vi "Write Device.vi"(8 "error in":errorcluster, 10 "Device":string, 11 "Config in":refnum<class "Config.lvclass">) -> (0 "error out":errorcluster, 3 "Config out":refnum<class "Config.lvclass">)   [LabVIEW 2023, in "Config.lvlib" / "Config.lvclass"]
doc: "Select device from list of devices and read all key labels and values for the device"
uses:
  Config.lvclass
  Config.lvclass/Config.ctl
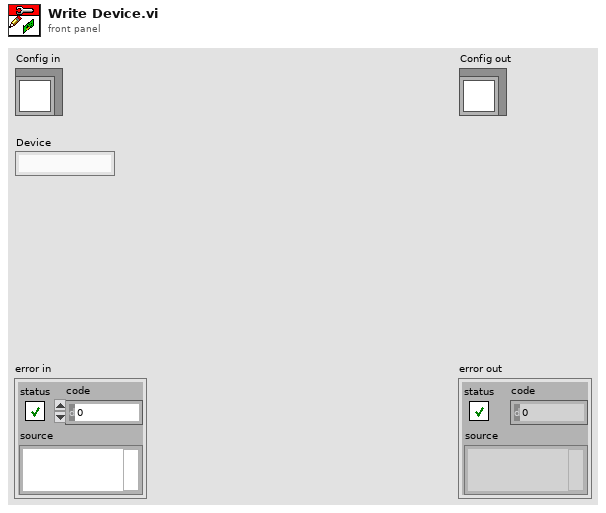
[diagram p1: front panel]
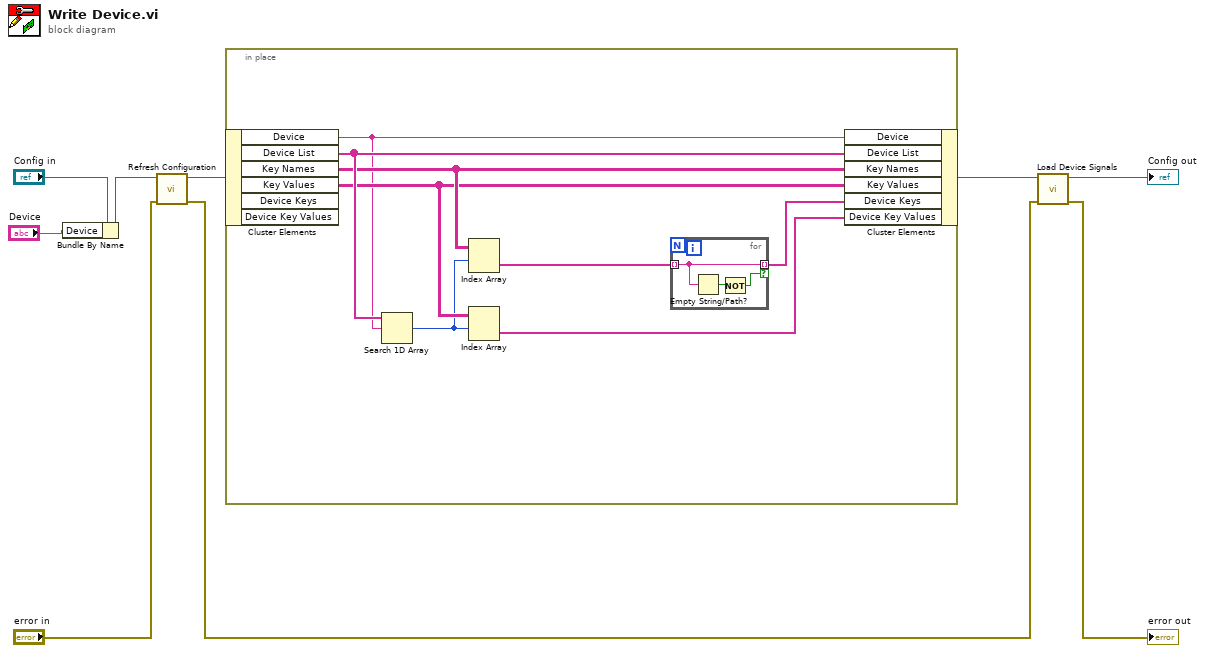
[diagram p0: block diagram]
diagram:
  n1 = Bundle By Name(cluster="Config in", "Device"="Device") -> (w7:refnum<class "Config.lvclass">)
  n2 = call "Refresh Configuration.vi"("error in"="error in", "Config in"=w7) -> ("error out"=w2:errorcluster, "Config out"=w6:refnum<class "Config.lvclass">)  [unwired: 8 in]
  n3 = in-place {
    n4 = in-place-cluster #1(w6) -> ("Device"=w11:string, "Device List"=w17:string[], "Key Names"=w16:string[][], "Key Values"=w15:string[][])  [unwired: 2 out]
    n5 = Search 1D Array(1D array=w17, element=w11) -> (index of element=w14:i32)  [unwired: 1 in]
    n6 = Index Array(array=w16, index (row)=w14) -> (element=w13:string[])  [unwired: 1 in]
    n7 = Index Array(array=w15, index (row)=w14) -> (element=w10:string[])  [unwired: 1 in]
    n8 = for {
      tunnel: w13 -> [w18] mode=indexing
      tunnel: [w18] -> w12 mode=indexing if=w19
      n9 = Empty String/Path?(string/path=w18) -> (empty?=w20:bool)
      n10 = Not(x=w20) -> (.not. x?=w19:bool)
    }
    n11 = in-place-cluster #1("Device"=w11, "Device List"=w17, "Key Names"=w16, "Key Values"=w15, "Device Keys"=w12, "Device Key Values"=w10) -> (w4:refnum<class "Config.lvclass">)
  }
  n12 = call "Load Device Signals.vi"("error in"=w2, "Config in"=w4) -> ("error out"=→"error out":errorcluster, "Config out"=→"Config out":refnum<class "Config.lvclass">)  [unwired: 8 in]
